vi "Motors Reset.vi"(2 "error in":errorcluster, 3 "VISA in":refnum<visa-resource-name>="COM7") -> (0 "error out":errorcluster, 1 "VISA out":refnum<visa-resource-name>)   [LabVIEW 2018]
panel:
  out "read buffer 4":string
  out "read buffer 3":string
  out "read buffer 2":string
  out "read buffer 1":string
  in  "RS4":string="04RS"
  in  "RS3":string="03RS"
  in  "RS2":string="02RS"
  in  "RS1":string="01RS"
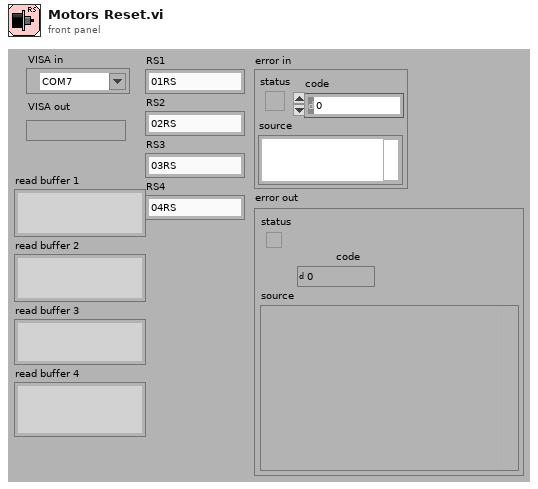
[diagram p1: front panel]
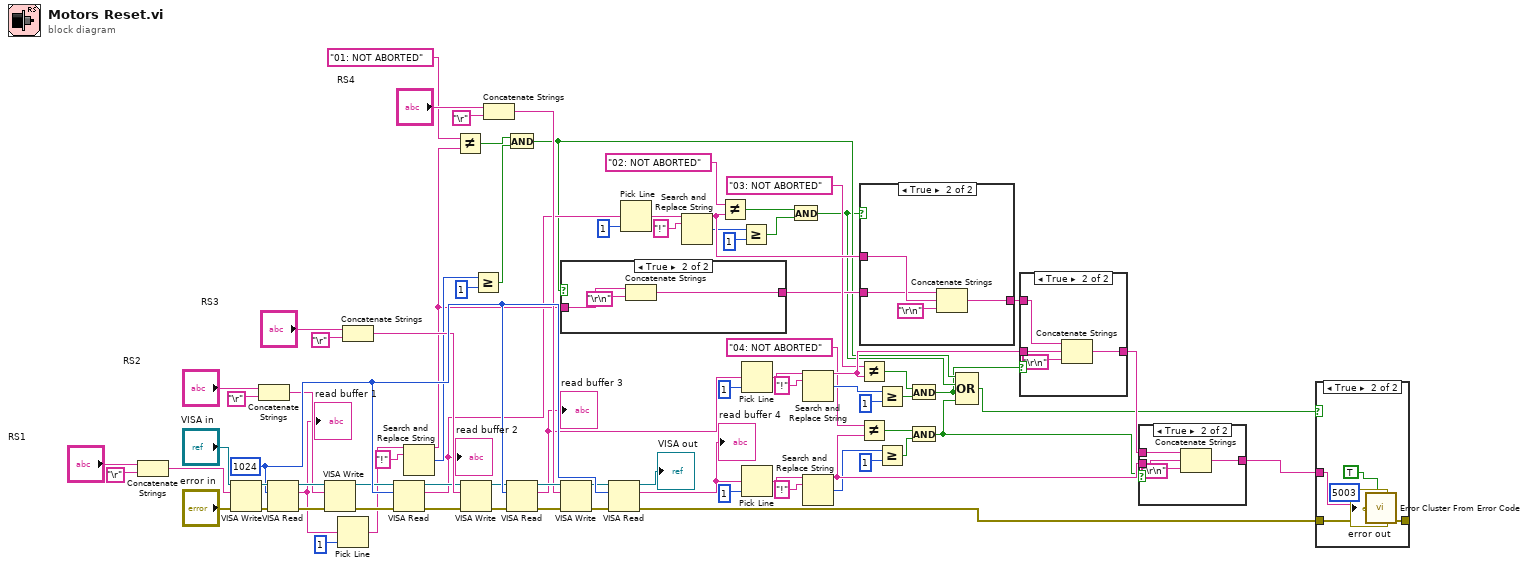
[diagram p0: block diagram]
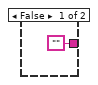
[diagram p3: hidden frame]
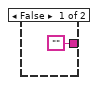
[diagram p4: hidden frame]
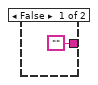
[diagram p5: hidden frame]
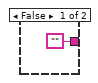
[diagram p6: hidden frame]
diagram:
  w75 = u32 1024 ("byte count")
  n1 = Concatenate Strings("RS1", "\r") -> (w79:string)
  n2 = VISA Write(VISA resource name="VISA in", write buffer=w79, error in (no error)="error in") -> (VISA resource name out=w76:refnum<visa-resource-name>, error out=w77:errorcluster)  [unwired: 1 out]
  n3 = Concatenate Strings("RS2", "\r") -> (w68:string)
  n4 = VISA Read(VISA resource name=w76, byte count=w75, error in (no error)=w77) -> (VISA resource name out=w74:refnum<visa-resource-name>, read buffer=w46:string, error out=w73:errorcluster)  [unwired: 1 out]
  "read buffer 1" <- w46
  n5 = VISA Write(VISA resource name=w74, write buffer=w68, error in (no error)=w73) -> (VISA resource name out=w72:refnum<visa-resource-name>, error out=w71:errorcluster)  [unwired: 1 out]
  n6 = Pick Line(multi-line string=w46, line index=1) -> (output string=w50:string)  [unwired: 1 in]
  n7 = Concatenate Strings("RS3", "\r") -> (w65:string)
  n8 = VISA Read(VISA resource name=w72, byte count=w75, error in (no error)=w71) -> (VISA resource name out=w63:refnum<visa-resource-name>, read buffer=w33:string, error out=w64:errorcluster)  [unwired: 1 out]
  "read buffer 2" <- w33
  n9 = Search and Replace String(input string=w50, search string="!") -> (result string=w44:string, number of replacements=w49:i32)  [unwired: 6 in, 2 out]
  n10 = Not Equal?(x="01: NOT ABORTED", y=w44) -> (x != y?=w6:bool)
  n11 = VISA Write(VISA resource name=w63, write buffer=w65, error in (no error)=w64) -> (VISA resource name out=w61:refnum<visa-resource-name>, error out=w62:errorcluster)  [unwired: 1 out]
  n12 = Greater Or Equal?(x=w49, y=1) -> (x >= y?=w45:bool)
  n13 = Concatenate Strings("RS4", "\r") -> (w55:string)
  n14 = And(x=w6, y=w45) -> (x .and. y?=w5:bool)
  n15 = VISA Read(VISA resource name=w61, byte count=w75, error in (no error)=w62) -> (VISA resource name out=w60:refnum<visa-resource-name>, read buffer=w23:string, error out=w59:errorcluster)  [unwired: 1 out]
  "read buffer 3" <- w23
  n16 = case shown="True" w5 {
    tunnel: w44 -> [_ w85]
    tunnel: ["" w84] -> w12
    frame False {
    }
    frame True {
      n17 = Concatenate Strings(w85, "\r\n") -> (w84:string)
    }
  }
  n18 = VISA Write(VISA resource name=w60, write buffer=w55, error in (no error)=w59) -> (VISA resource name out=w57:refnum<visa-resource-name>, error out=w58:errorcluster)  [unwired: 1 out]
  n19 = VISA Read(VISA resource name=w57, byte count=w75, error in (no error)=w58) -> (VISA resource name out=→"VISA out":refnum<visa-resource-name>, read buffer=w13:string, error out=w9:errorcluster)  [unwired: 1 out]
  "read buffer 4" <- w13
  n20 = Pick Line(multi-line string=w33, line index=1) -> (output string=w35:string)  [unwired: 1 in]
  n21 = Search and Replace String(input string=w35, search string="!") -> (result string=w40:string, number of replacements=w36:i32)  [unwired: 6 in, 2 out]
  n22 = Not Equal?(x="02: NOT ABORTED", y=w40) -> (x != y?=w42:bool)
  n23 = Greater Or Equal?(x=w36, y=1) -> (x >= y?=w39:bool)
  n24 = Pick Line(multi-line string=w23, line index=1) -> (output string=w31:string)  [unwired: 1 in]
  n25 = Pick Line(multi-line string=w13, line index=1) -> (output string=w15:string)  [unwired: 1 in]
  n26 = And(x=w42, y=w39) -> (x .and. y?=w4:bool)
  n27 = Search and Replace String(input string=w31, search string="!") -> (result string=w26:string, number of replacements=w30:i32)  [unwired: 6 in, 2 out]
  n28 = Search and Replace String(input string=w15, search string="!") -> (result string=w20:string, number of replacements=w16:i32)  [unwired: 6 in, 2 out]
  n29 = Not Equal?(x="03: NOT ABORTED", y=w26) -> (x != y?=w24:bool)
  n30 = Not Equal?(x="04: NOT ABORTED", y=w20) -> (x != y?=w22:bool)
  n31 = case shown="True" w4 {
    tunnel: w40 -> [_ w90]
    tunnel: ["" w89] -> w11
    tunnel: w12 -> [_ w87]
    frame False {
    }
    frame True {
      n32 = Concatenate Strings(w87, w90, "\r\n") -> (w89:string)
    }
  }
  n33 = Greater Or Equal?(x=w30, y=1) -> (x >= y?=w27:bool)
  n34 = Greater Or Equal?(x=w16, y=1) -> (x >= y?=w19:bool)
  n35 = And(x=w24, y=w27) -> (x .and. y?=w3:bool)
  n36 = And(x=w22, y=w19) -> (x .and. y?=w1:bool)
  n37 = Compound Arithmetic op=OR(w5, w4, w3, w1) -> (w2:bool)
  n38 = case shown="True" w3 {
    tunnel: w26 -> [_ w95]
    tunnel: ["" w94] -> w10
    tunnel: w11 -> [_ w92]
    frame False {
    }
    frame True {
      n39 = Concatenate Strings(w92, w95, "\r\n") -> (w94:string)
    }
  }
  n40 = case shown="True" w1 {
    tunnel: w20 -> [_ w100]
    tunnel: ["" w99] -> w7
    tunnel: w10 -> [_ w97]
    frame False {
    }
    frame True {
      n41 = Concatenate Strings(w97, w100, "\r\n") -> (w99:string)
    }
  }
  n42 = case shown="True" w2 {
    tunnel: w9 -> [w101 w106]
    tunnel: [w101 w105] -> w8
    tunnel: w7 -> [_ w104]
    frame False {
    }
    frame True {
      n43 = call <vilib>:"Error Cluster From Error Code.vi"("show call chain? (False)"=TRUE, "error in (no error)"=w106, "error message (\"\")"=w104, "error code (0)"=5003) -> ("error out"=w105:errorcluster)  [unwired: 5 in]
    }
  }
  "error out" <- w8
